vi "Xylo_Final_Melodia.vi"() -> ()   [LabVIEW 2018]
panel:
  in  "Open Button":bool
  in  "Save As Button":bool
  out "tableauRythme":u8[](array[numeric])
  in  "Rythme Choix":string(combo)
  in  "RESET Button":bool
  out "tableauNotes":u8[](array[numeric])
  in  "stop":bool
  out "Numeric":i32
  in  "Array":bool[](array[boolean])=[FALSE, FALSE, FALSE, FALSE, FALSE, FALSE, FALSE, FALSE] caption="Clavier"
  out "Messure Musicale":dbl(graph)
  in  "File Path Control 2":path
  in  "Save Button":bool
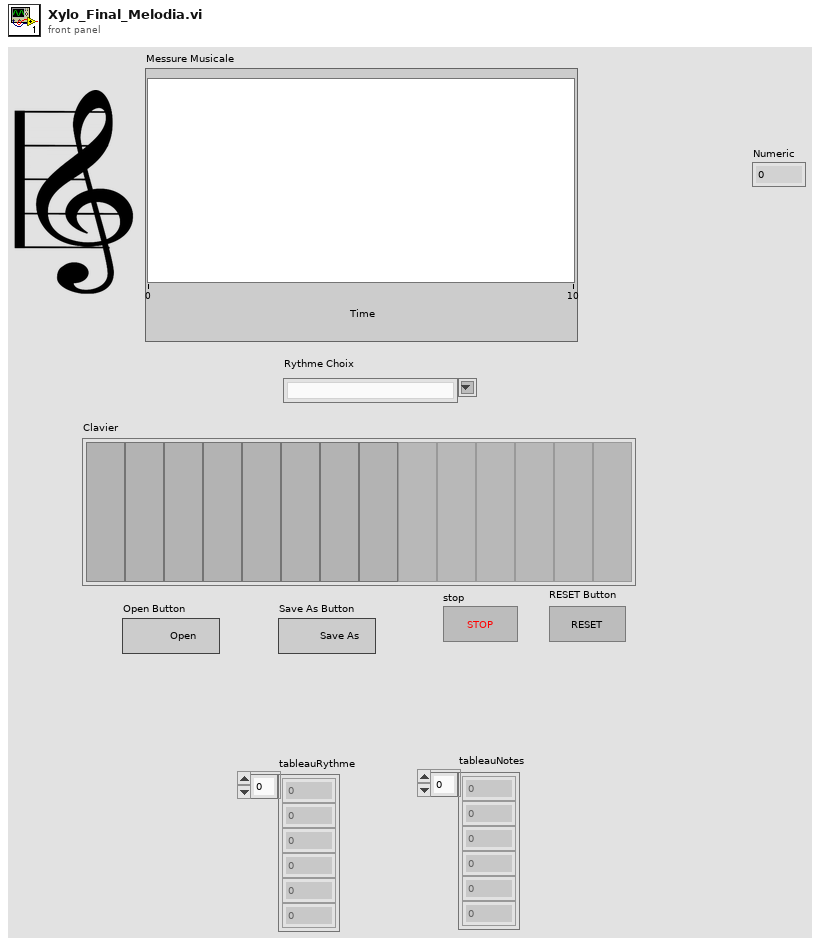
[diagram p1: front panel]
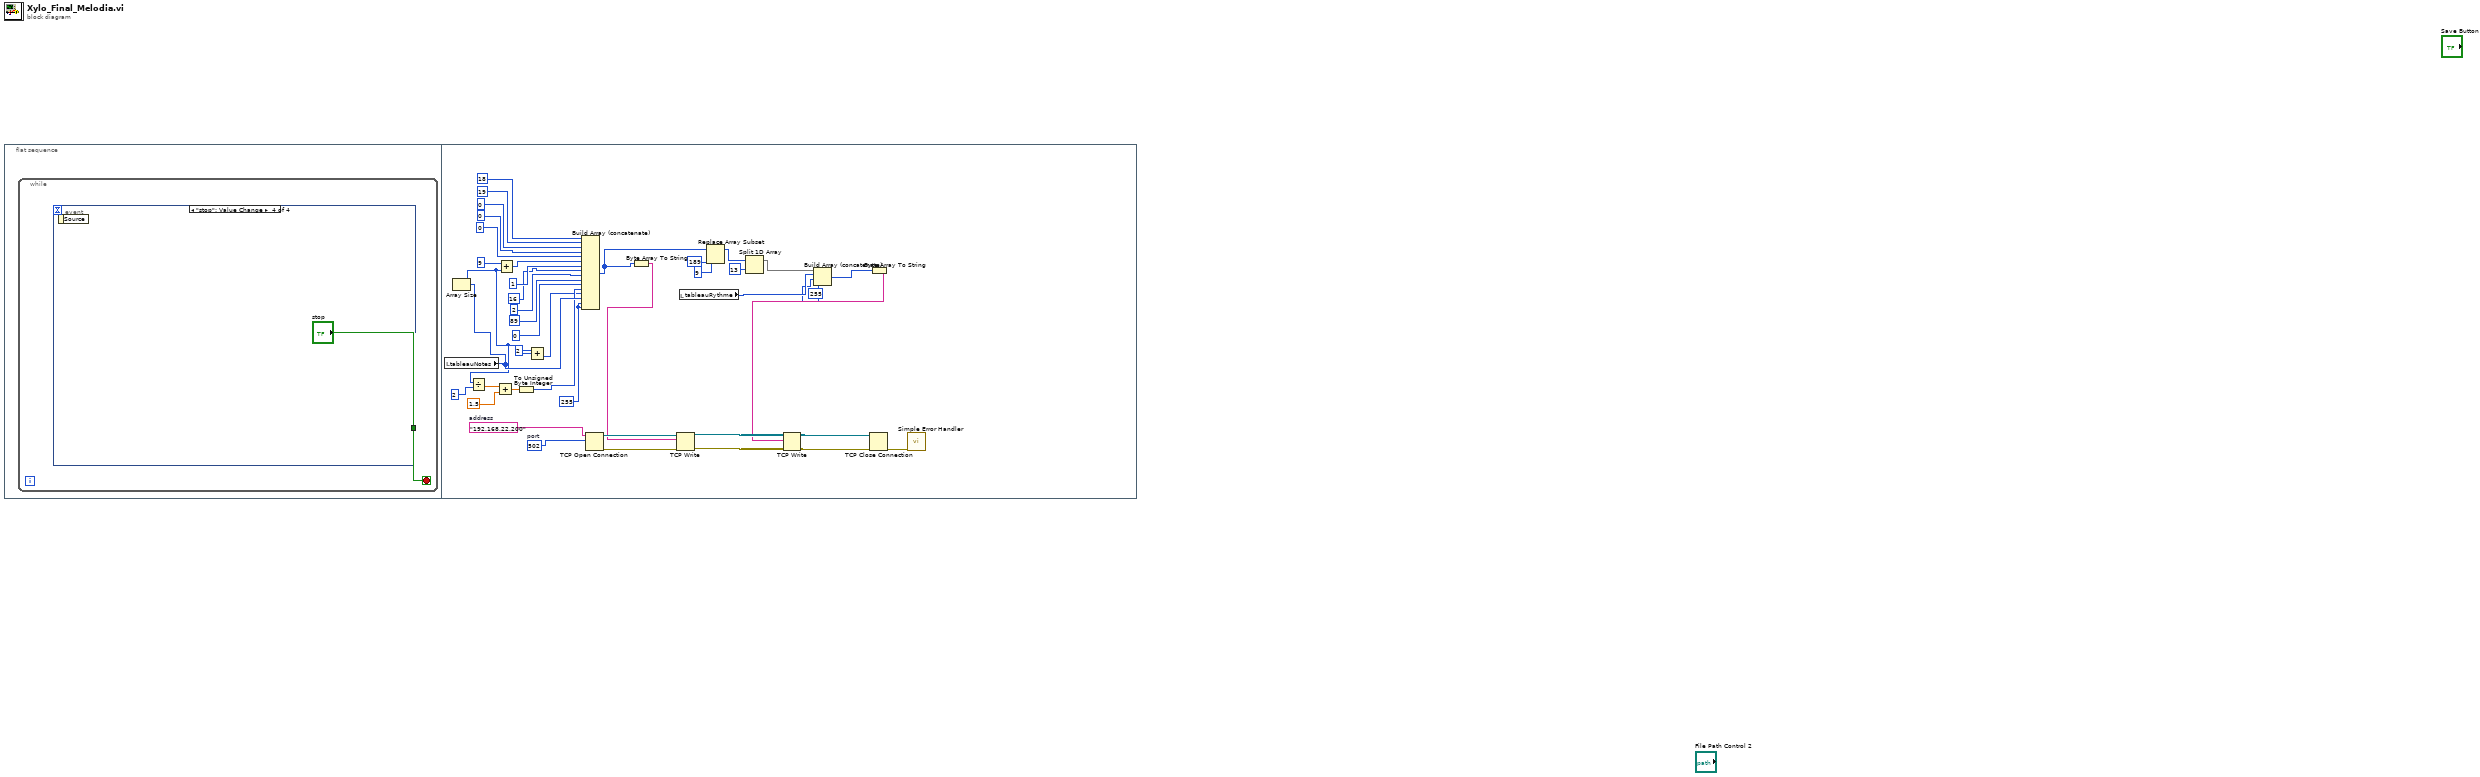
[diagram p0: block diagram]
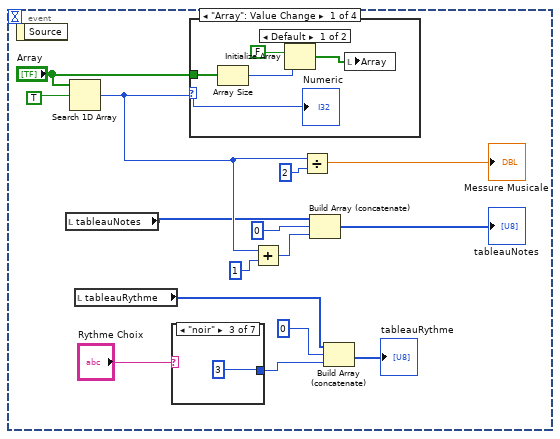
[diagram p2: hidden frame]
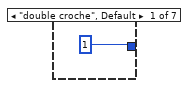
[diagram p3: hidden frame]
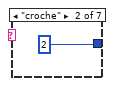
[diagram p4: hidden frame]
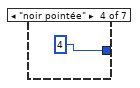
[diagram p5: hidden frame]
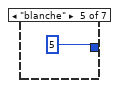
[diagram p6: hidden frame]
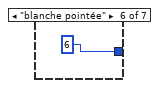
[diagram p7: hidden frame]
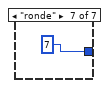
[diagram p8: hidden frame]
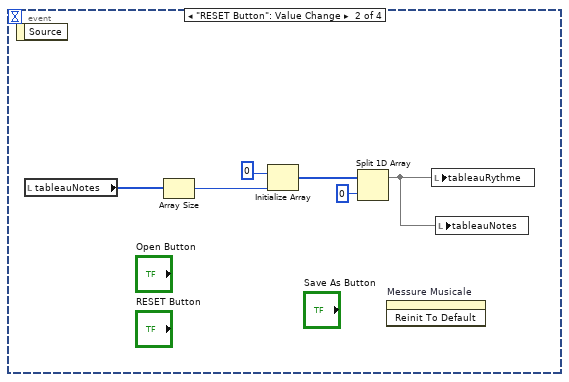
[diagram p10: hidden frame]
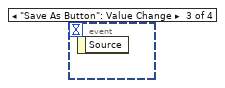
[diagram p11: hidden frame]
diagram:
  n1 = flat-sequence {
    frame #0 {
      n2 = while {
        stop <- w1 stop-if-true
        n3 = event shown="[3] \"stop\": Value Change" {
          selector: _ -> [_ _ _ _]
          dyn-events: _ -> [_ _ _ _]
          timeout: _ -> [_ _ _ _]
          tunnel: [_ _ _ "stop"] -> w1
          event "Array": Value Change {
            n4 = event-data() -> ()  [unwired: 1 in, 1 out]
            n5 = local read "tableauNotes"() -> (w10:u8[])
            n6 = Search 1D Array(1D array="Array", element=TRUE) -> (index of element=w12:i32)  [unwired: 1 in]
            n7 = local read "tableauRythme"() -> (w2:u8[])
            n8 = case shown="\"noir\"" "Rythme Choix" {
              tunnel: [1 2 3 4 5 6 7] -> w4
              frame "double croche", Default {
              }
              frame "croche" {
              }
              frame "noir" {
              }
              frame "noir pointée" {
              }
              frame "blanche" {
              }
              frame "blanche pointée" {
              }
              frame "ronde" {
              }
            }
            n9 = case shown="Default" w12 {
              selector: w12 -> [w25 _]
              tunnel: "Array" -> [w26 _]
              frame Default {
                n10 = Array Size(array=w26) -> (size(s)=w28:i32)
                n11 = Initialize Array(FALSE ("element"), w28) -> (w24:bool[])
                n12 = local write "Array"(w24) -> ()
                "Numeric" <- w25
              }
              frame -1 {
              }
            }
            n13 = Add(x=w12, y=1) -> (x+y=w9:i32)
            n14 = Divide(x=w12, y=2 ("Numeric")) -> (x/y=→"Messure Musicale":dbl)
            n15 = Build Array (concatenate)(w10, 0 ("element"), w9) -> (→"tableauNotes":i32[])
            n16 = Build Array (concatenate)(w2, 0 ("element"), w4) -> (→"tableauRythme":i32[])
          }
          event "RESET Button": Value Change {
            n17 = event-data() -> ()  [unwired: 1 in, 1 out]
            n18 = local read "tableauNotes"() -> (w33:u8[])
            n19 = Array Size(array=w33) -> (size(s)=w32:i32)
            n20 = Initialize Array(u8 0 ("element"), w32) -> (w31:u8[])
            n21 = Split 1D Array(array=w31, index=0) -> (first subarray=w29:u8[])  [unwired: 1 out]
            n22 = invoke on="Messure Musicale" class="WFChart (strict)" method="Reinit To Default"() -> ()  [unwired: 3 in, 3 out]
            n23 = local write "tableauRythme"(w29) -> ()
            n24 = local write "tableauNotes"(w29) -> ()
          }
          event "Save As Button": Value Change {
            n25 = event-data() -> ()  [unwired: 1 in, 1 out]
          }
          event "stop": Value Change {
            n26 = event-data() -> ()  [unwired: 1 in, 1 out]
          }
        }
      }
    }
    frame #1 {
      w38 = 255
      w39 = 255
      w75 = "192.168.22.200"  # address
      w76 = 502  # port
      n27 = local read "tableauNotes"() -> (w48:u8[])
      n28 = Array Size(array=w48) -> (size(s)=w40:i32)
      n29 = Divide(x=w40, y=2) -> (x/y=w60:dbl)
      n30 = Add(x=w60, y=1.5) -> (x+y=w61:dbl)
      n31 = Add(x=9, y=w40) -> (x+y=w64:i32)
      n32 = To Unsigned Byte Integer(number=w61) -> (unsigned 8bit integer=w41:u8)
      n33 = Add(x=2, y=w40) -> (x+y=w37:i32)
      n34 = Build Array (concatenate)(18, 19, 0, 0, 0, w64, 1, 16, 2, 89, 0, w41, w37, w48, w39, w39) -> (w43:i32[])
      n35 = TCP Open Connection(address=w75, remote port or service name=w76) -> (connection ID=w50:refnum<k5>, error out=w49:errorcluster)  [unwired: 3 in]
      n36 = Byte Array To String(unsigned byte array=w43) -> (string=w42:string)
      n37 = TCP Write(connection ID=w50, data in=w42, error in (no error)=w49) -> (connection ID out=w74:refnum<k5>, error out=w73:errorcluster)  [unwired: 1 in, 1 out]
      n38 = local read "tableauRythme"() -> (w47:u8[])
      n39 = Replace Array Subset(array=w43, new element=189 ("new element/subarray"), index=9) -> (w55:i32[])
      n40 = Split 1D Array(array=w55, index=13) -> (first subarray=w57:i32[])  [unwired: 1 out]
      n41 = Build Array (concatenate)(w57, w47, w38, w38) -> (w56:i32[])
      n42 = Byte Array To String(unsigned byte array=w56) -> (string=w46:string)
      n43 = TCP Write(connection ID=w74, data in=w46, error in (no error)=w73) -> (connection ID out=w71:refnum<k5>, error out=w72:errorcluster)  [unwired: 1 in, 1 out]
      n44 = TCP Close Connection(connection ID=w71, error in (no error)=w72) -> (error out=w77:errorcluster)  [unwired: 1 in, 1 out]
      n45 = call <vilib>:"Simple Error Handler.vi"("error in (no error)"=w77) -> ()  [unwired: 4 in, 5 out]
    }
  }
